vi "PDCConvertShutter.vi"(10 "ShutterValue":u16, 11 "ShutterList":string[](array[string])) -> (3 "ShutterSpeed":u32)   [LabVIEW 2015]
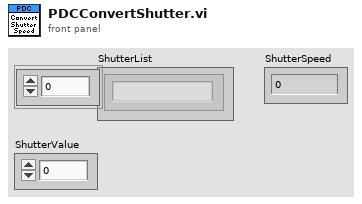
[diagram p1: front panel]
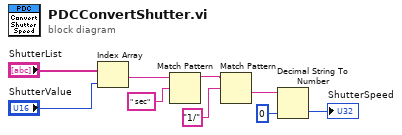
[diagram p0: block diagram]
diagram:
  n1 = Index Array(array="ShutterList", index="ShutterValue") -> (element=w6:string)
  n2 = Match Pattern(string=w6, regular expression=" sec") -> (before substring=w3:string)  [unwired: 4 out]
  n3 = Match Pattern(string=w3, regular expression="1/") -> (after substring=w1:string)  [unwired: 4 out]
  n4 = Decimal String To Number(string=w1, default (0L)=u32 0 ("デフォルト (0 I32)")) -> (number=→"ShutterSpeed":u32)  [unwired: 2 out]
